vi "Add hyperlink.vi"(7 "overwrite?":bool=TRUE, 9 "error in (no error)":errorcluster, 10 "URL":string, 11 "Properties":refnum<class "Properties.lvclass">) -> (1 "error out":errorcluster, 3 "Properties":refnum<class "Properties.lvclass">)   [LabVIEW 2013, in "Caraya.lvlib" / "Properties.lvclass"]
uses:
  Properties.lvclass
  Properties.lvclass/Properties.ctl
  Test Manager Message KVP/TestManagerMsg.KVP.lvclass
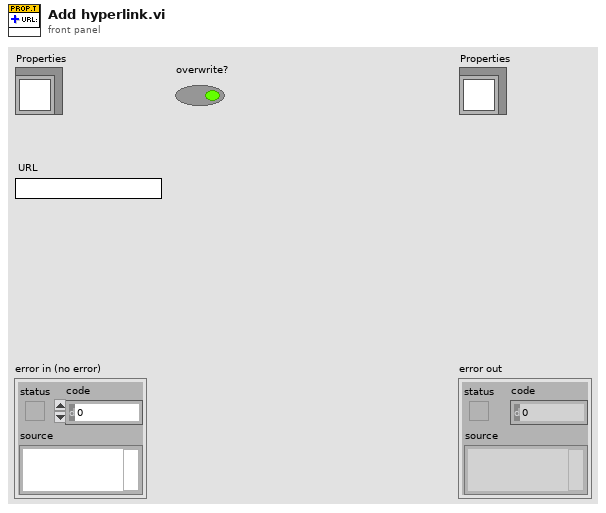
[diagram p1: front panel]
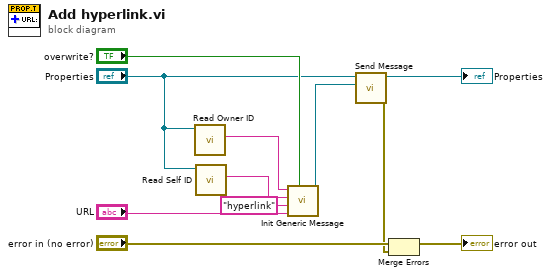
[diagram p0: block diagram]
diagram:
  n1 = call "Read Owner ID.vi"("Properties in"="Properties") -> ("owner-id"=w5:string)  [unwired: 9 in, 1 out]
  n2 = call "Read Self ID.vi"("Properties in"="Properties") -> ("self-id"=w6:string)  [unwired: 9 in, 1 out]
  n3 = call "Init Generic Message.vi"("overwrite?"="overwrite?", "value"="URL", "key"="hyperlink", "self-id"=w6, "owner-id"=w5) -> ("Message"=w2:refnum<class "TestManagerMsg.lvclass">)  [unwired: 6 in]
  n4 = call "Send Message.vi"("TestManagerMsg"=w2, "Properties in"="Properties") -> ("error out"=w1:errorcluster, "Properties out"=→"Properties":refnum<class "Properties.lvclass">)  [unwired: 8 in]
  n5 = Merge Errors("error in (no error)", w1) -> (→"error out":errorcluster)
